vi "StarttoGoalLine.vi"(8 "y1":i32, 9 "x1":i32, 10 "y0":i32, 11 "x0":i32) -> (2 "y Line coords":i32[](array[numeric]), 3 "x Line coords":i32[](array[numeric]))   [LabVIEW 2013, in "RVCLibrary_Bug2.lvclass"]
uses:
  RVCLibrary_Bug2.lvclass
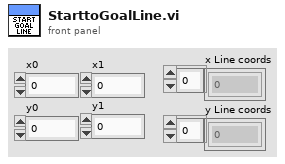
[diagram p1: front panel]
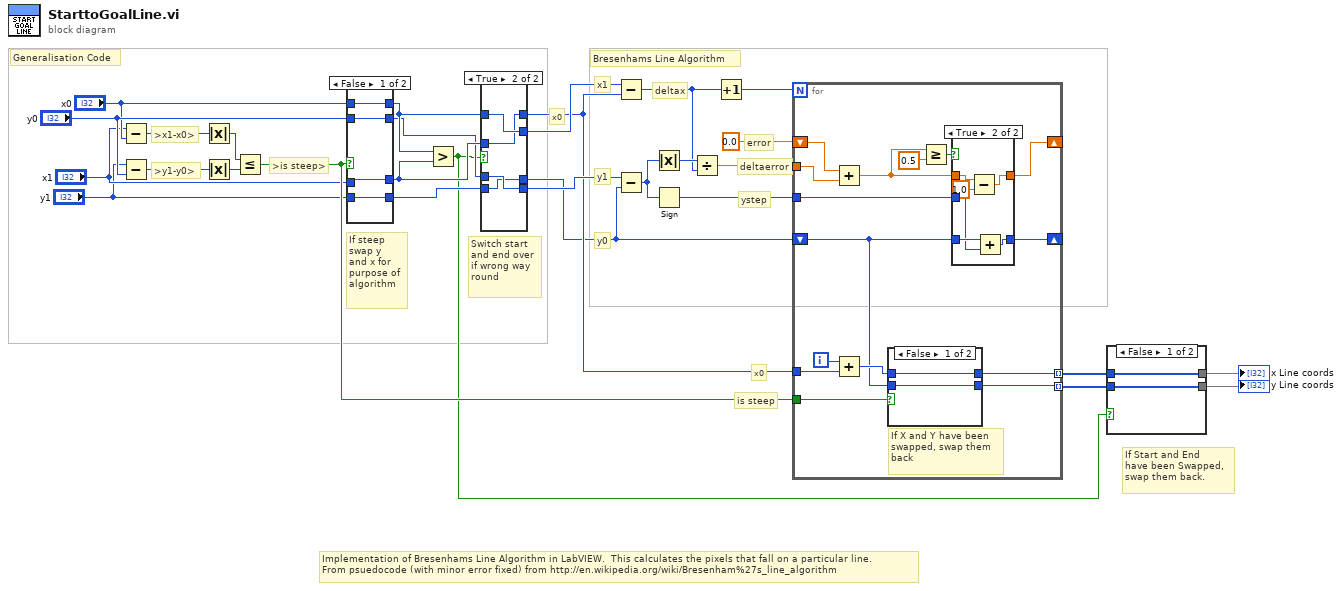
[diagram p0: block diagram]
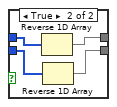
[diagram p2: hidden frame]
diagram:
  # "Bresenhams Line Algorithm"
  # "If Start and End\nhave been Swapped,\nswap them back."
  # "Implementation of Bresenhams Line Algorithm in LabVIEW.  This calculates the pixels that fall on a particular line.\nFrom psuedocode (with minor error fixed) from http://en.wikipedia.org/wiki/Bresenham%27s_line_algorithm"
  # "Switch start\nand end over\nif wrong way\nround"
  # "If steep\nswap y\nand x for\npurpose of\nalgorithm"
  # "is steep"
  # "x0"
  # "Generalisation Code"
  # "y0"
  # "deltaerror"
  # "error"
  # "ystep"
  # "deltax"
  # "y1"
  # "x1"
  # "x0"
  # ">is steep>"
  # ">y1-y0>"
  # ">x1-x0>"
  n1 = Subtract(x="x1", y="x0") -> (x-y=w29:i32)
  n2 = Subtract(x="y1", y="y0") -> (x-y=w28:i32)
  n3 = Absolute Value(x=w29) -> (abs(x)=w26:i32)
  n4 = Absolute Value(x=w28) -> (abs(x)=w27:i32)
  n5 = Less Or Equal?(x=w26, y=w27) -> (x <= y?=w12:bool)
  n6 = case shown="False" w12 {
    tunnel: "x0" -> [w33 w37]
    tunnel: "x1" -> [w32 w36]
    tunnel: "y0" -> [w31 w35]
    tunnel: "y1" -> [w30 w34]
    tunnel: [w31 w37] -> w23
    tunnel: [w30 w36] -> w22
    tunnel: [w33 w35] -> w25
    tunnel: [w32 w34] -> w24
    frame False {
    }
    frame True {
    }
  }
  n7 = Greater?(x=w25, y=w24) -> (0:w9:bool)
  n8 = case shown="True" w9 {
    tunnel: w25 -> [w41 w45]
    tunnel: w24 -> [w40 w44]
    tunnel: w23 -> [w39 w43]
    tunnel: w22 -> [w38 w42]
    tunnel: [w41 w44] -> w17
    tunnel: [w40 w45] -> w21
    tunnel: [w39 w42] -> w14
    tunnel: [w38 w43] -> w20
    frame False {
    }
    frame True {
    }
  }
  n9 = Subtract(x=w21, y=w17) -> (x-y=w11:i32)
  n10 = Subtract(x=w20, y=w14) -> (x-y=w18:i32)
  n11 = Absolute Value(x=w18) -> (abs(x)=w19:i32)
  n12 = Sign(1:w18) -> (0:w13:i32)
  n13 = Divide(x=w19, y=w11) -> (x/y=w15:dbl)
  n14 = Increment(x=w11) -> (x+1=w10:i32)
  n15 = for {
    N: w10 -> [_]
    tunnel: w17 -> [w59]
    shift-right: [w49] -> _
    shift-left: 0.0 -> [w50]
    tunnel: w15 -> [w58]
    tunnel: w13 -> [w52]
    tunnel: w12 -> [w57]
    shift-right: [w51] -> _
    shift-left: w14 -> [w53]
    tunnel: [w47] -> w4 mode=indexing
    tunnel: [w46] -> w3 mode=indexing
    i -> [w60]
    # "If X and Y have been\nswapped, swap them\nback"
    n16 = Add(x=w50, y=w58) -> (x+y=w48:dbl)
    n17 = Add(x=w60, y=w59) -> (x+y=w56:i32)
    n18 = case shown="False" w57 {
      tunnel: w53 -> [w69 w72]
      tunnel: [w70 w72] -> w47
      tunnel: w56 -> [w70 w71]
      tunnel: [w69 w71] -> w46
      frame False {
      }
      frame True {
      }
    }
    n19 = Greater Or Equal?(x=w48, y=0.5) -> (x >= y?=w55:bool)
    n20 = case shown="True" w55 {
      tunnel: w53 -> [w61 w68]
      tunnel: w52 -> [_ w65]
      tunnel: [w61 w67] -> w51
      tunnel: w48 -> [w62 w66]
      tunnel: [w62 w64] -> w49
      frame False {
      }
      frame True {
        n21 = Subtract(x=w66, y=1.0) -> (x-y=w64:dbl)
        n22 = Add(x=w68, y=w65) -> (x+y=w67:i32)
      }
    }
  }
  n23 = case shown="False" w9 {
    tunnel: [w74 w78] -> w2
    tunnel: w4 -> [w74 w77]
    tunnel: w3 -> [w73 w76]
    tunnel: [w73 w75] -> w1
    frame False {
    }
    frame True {
      n24 = Reverse 1D Array(array=w77) -> (reversed array=w78:i32[])
      n25 = Reverse 1D Array(array=w76) -> (reversed array=w75:i32[])
    }
  }
  "x Line coords" <- w2
  "y Line coords" <- w1
